vi "Configure Output Impedance.vi"(8 "error in (no error)":errorcluster, 9 "Impedance (0: 50 Ohms)":u16(ring) items=["50 Ohms", "High Impedance"], 10 "Channel (1:Channel 1)":i32(ring)=1 items=["Channel 1"=1, "Channel 2"=2], 11 "VISA resource name":refnum<visa-resource-name>) -> (0 "error out":errorcluster, 3 "VISA resource name out":refnum<visa-resource-name>)   [LabVIEW 2022 SP3, in "Siglent SDG X Series.lvlib"]
doc: "Configures the output impedance of the selected channel."
uses:
  Siglent SDG X Series.lvlib
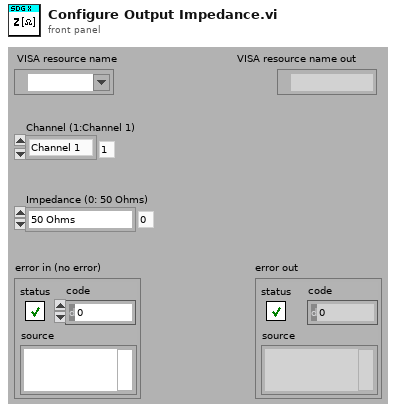
[diagram p1: front panel]
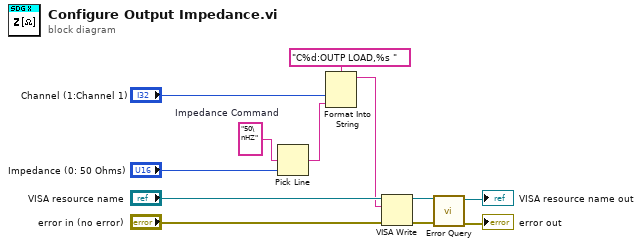
[diagram p0: block diagram]
diagram:
  w10 = "50\nHZ"  # Impedance Command
  n1 = Pick Line(multi-line string=w10, line index="Impedance (0: 50 Ohms)") -> (output string=w7:string)  [unwired: 1 in]
  n2 = Format Into String(format string="C%d:OUTP LOAD,%s ", "Channel (1:Channel 1)", w7) -> (resulting string=w6:string)  [unwired: 2 in, 1 out]
  n3 = VISA Write(VISA resource name="VISA resource name", write buffer=w6, error in (no error)="error in (no error)") -> (VISA resource name out=w3:refnum<visa-resource-name>, error out=w4:errorcluster)  [unwired: 1 out]
  n4 = call "Error Query.vi"("error in (no error)"=w4, "VISA resource name"=w3) -> ("error out"=→"error out":errorcluster, "VISA resource name out"=→"VISA resource name out":refnum<visa-resource-name>)  [unwired: 6 in, 2 out]
